vi "Page_Hardware_Write.vi"(6 "ctlReferences":T1, 8 "error in (no error)":errorcluster, 11 "Class in":refnum<class "Installer.lvclass">) -> (0 "error out":errorcluster, 3 "Class out":refnum<class "Installer.lvclass">)   [LabVIEW 2020, in "Installer.lvclass"]
uses:
  <vilib>/AppBuilder/IB_Classes/Installer/Installer.lvclass
  <resource>/Framework/Providers/Builds/Installer/Pages/controls/IB_UI_Page_Hardware_References.ctl
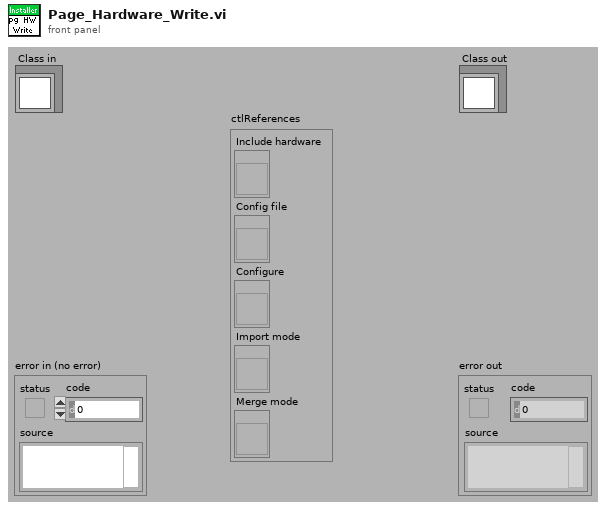
[diagram p1: front panel]
types:
  T1 = typedef "IB_UI_Page_Hardware_References.ctl" = cluster{"Include hardware":refnum<vi>, "Config file":refnum<vi>, "Configure":refnum<vi>, "Import mode":refnum<vi>, "Merge mode":refnum<vi>}
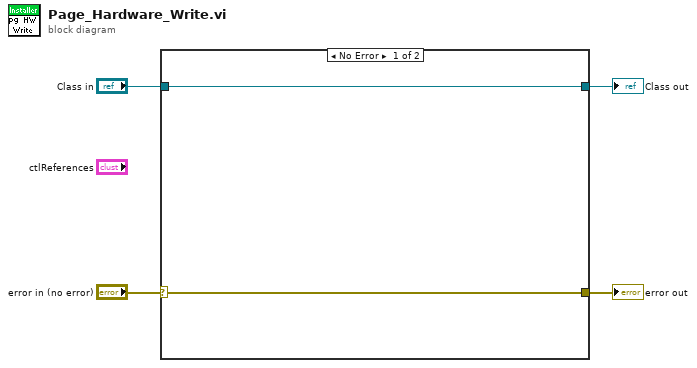
[diagram p0: block diagram]
diagram:
  n1 = case shown="No Error" "error in (no error)" {
    selector: "error in (no error)" -> [w6 w8]
    tunnel: [w6 w8] -> w3
    tunnel: [w5 w7] -> w1
    tunnel: "Class in" -> [w5 w7]
    frame No Error {
    }
    frame Error {
    }
  }
  "error out" <- w3
  "Class out" <- w1
